vi "Initialize.vi"(7 "Channel Name":string="Setpoint.ch%d.SP", 8 "error in":errorcluster, 9 "Number of Channels":u32=1, 10 "Instance Name":string="PluginName", 11 "Current Limit in":refnum<class "Current Limit.lvclass">) -> (0 "error out":errorcluster caption="error in", 3 "Current Limit out":refnum<class "Current Limit.lvclass">)   [LabVIEW 2023, in "Current Limit.lvclass"]
uses:
  Current Limit.lvclass
  Parents/Limit/Limit.lvclass
  Current Limit.lvclass/Current Limit.ctl
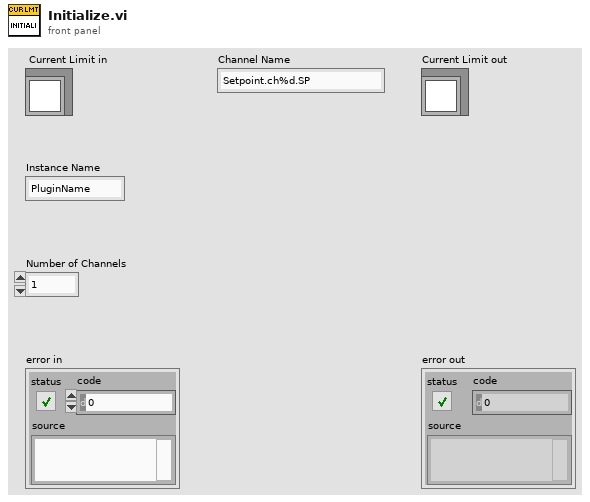
[diagram p1: front panel]
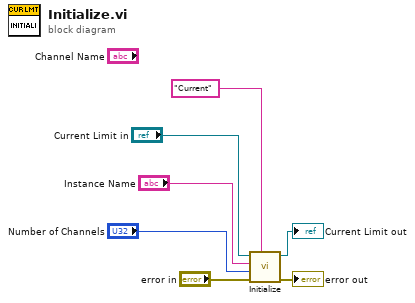
[diagram p0: block diagram]
diagram:
  n1 = call-parent "Initialize.vi"("LimitMAX.ch%d.SP"="Current", "error in"="error in", "Number of Channels"="Number of Channels", "Instance Name"="Instance Name", "Limit in"="Current Limit in") -> ("error out"=→"error out":errorcluster, "Limit out"=→"Current Limit out":refnum<class "Current Limit.lvclass">)  [unwired: 5 in]
